vi "Get Event HMI Autotest.vi"(8 "error in (no error)":errorcluster caption="entrée d'erreur (pas d'erreur)", 11 "Actor_Autotest en entrée":refnum<class "Actor_Autotest.lvclass">) -> (0 "error out":errorcluster caption="sortie d'erreur", 2 "Event Autotest":refnum<user-event>, 3 "Actor_Autotest en sortie":refnum<class "Actor_Autotest.lvclass">)   [LabVIEW 2020, in "Library Core.lvlib" / "Actor_Autotest.lvlib" / "Actor_Autotest.lvclass"]
uses:
  Actor_Autotest.lvclass
  Instrument/Instrument (Default)/Class Instrument (Default).lvclass
  Commun VI/TypeDef/Commande Popup autotest/Commande element autotest.ctl
  Actor_Autotest.lvclass/Actor_Autotest.ctl
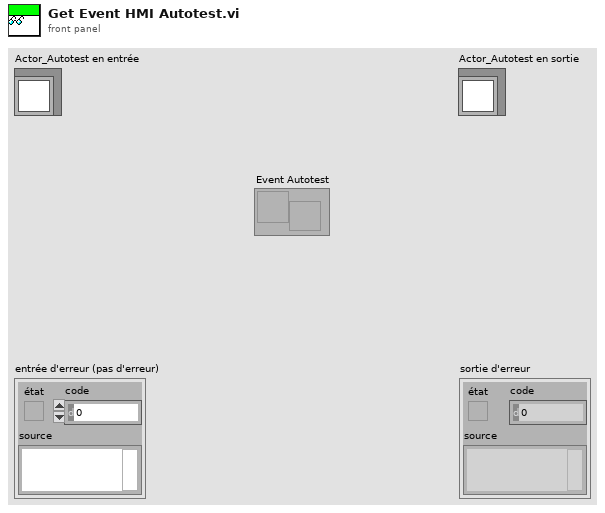
[diagram p1: front panel]
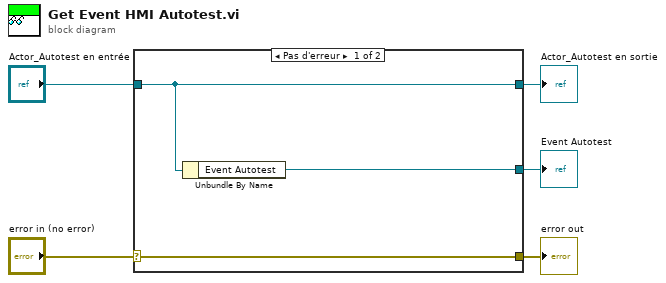
[diagram p0: block diagram]
diagram:
  n1 = case shown="Pas d'erreur" "error in (no error)" {
    selector: "error in (no error)" -> [w8 w9]
    tunnel: [w8 w9] -> w4
    tunnel: [w7 w10] -> w2
    tunnel: "Actor_Autotest en entrée" -> [w7 w10]
    tunnel: [w6 _] -> w1
    frame No Error {
      n2 = Unbundle By Name(w7) -> ("Event Autotest"=w6:refnum<user-event>)
    }
    frame Error {
    }
  }
  "error out" <- w4
  "Actor_Autotest en sortie" <- w2
  "Event Autotest" <- w1
